vi "initialize.vi"(7 "parameters":string[][](array[string]), 8 "error in":errorcluster, 10 "server id":i32, 11 "message json":string) -> (0 "error out":errorcluster, 3 "response":string)   [LabVIEW 2025, in "MCP Server.lvlib"]
uses:
  MCP Server.lvlib
  098ae85c-509d-4dd3-b755-49cb06aac0fc.vi
  <vilib>/JDP Science/JSONtext/Variant to JSON Text.vi
  <vilib>/JDP Science/JSONtext/LVClass Serializer/JSONtext LVClass Serializer.lvclass
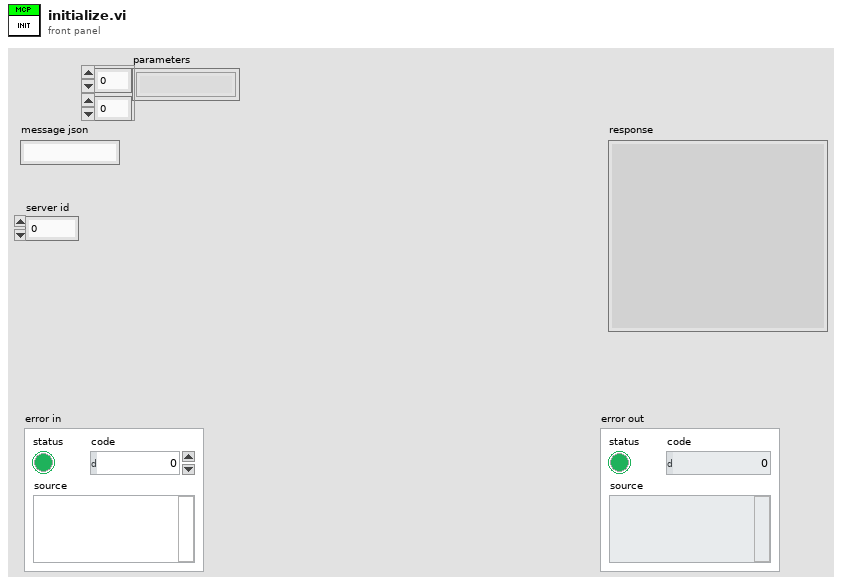
[diagram p1: front panel]
types:
  T1 = cluster{"protocolVersion":string, "capabilities":cluster{"tools":cluster{"listChanged":bool}, "prompts":cluster{"listChanged":bool}, "resources":cluster{"subscribe":bool, "listChanged":bool}}, "serverInfo":cluster{"name":string, "version":string, "additionalDetails":cluster{"labviewVersion":string, "platform":string}}}
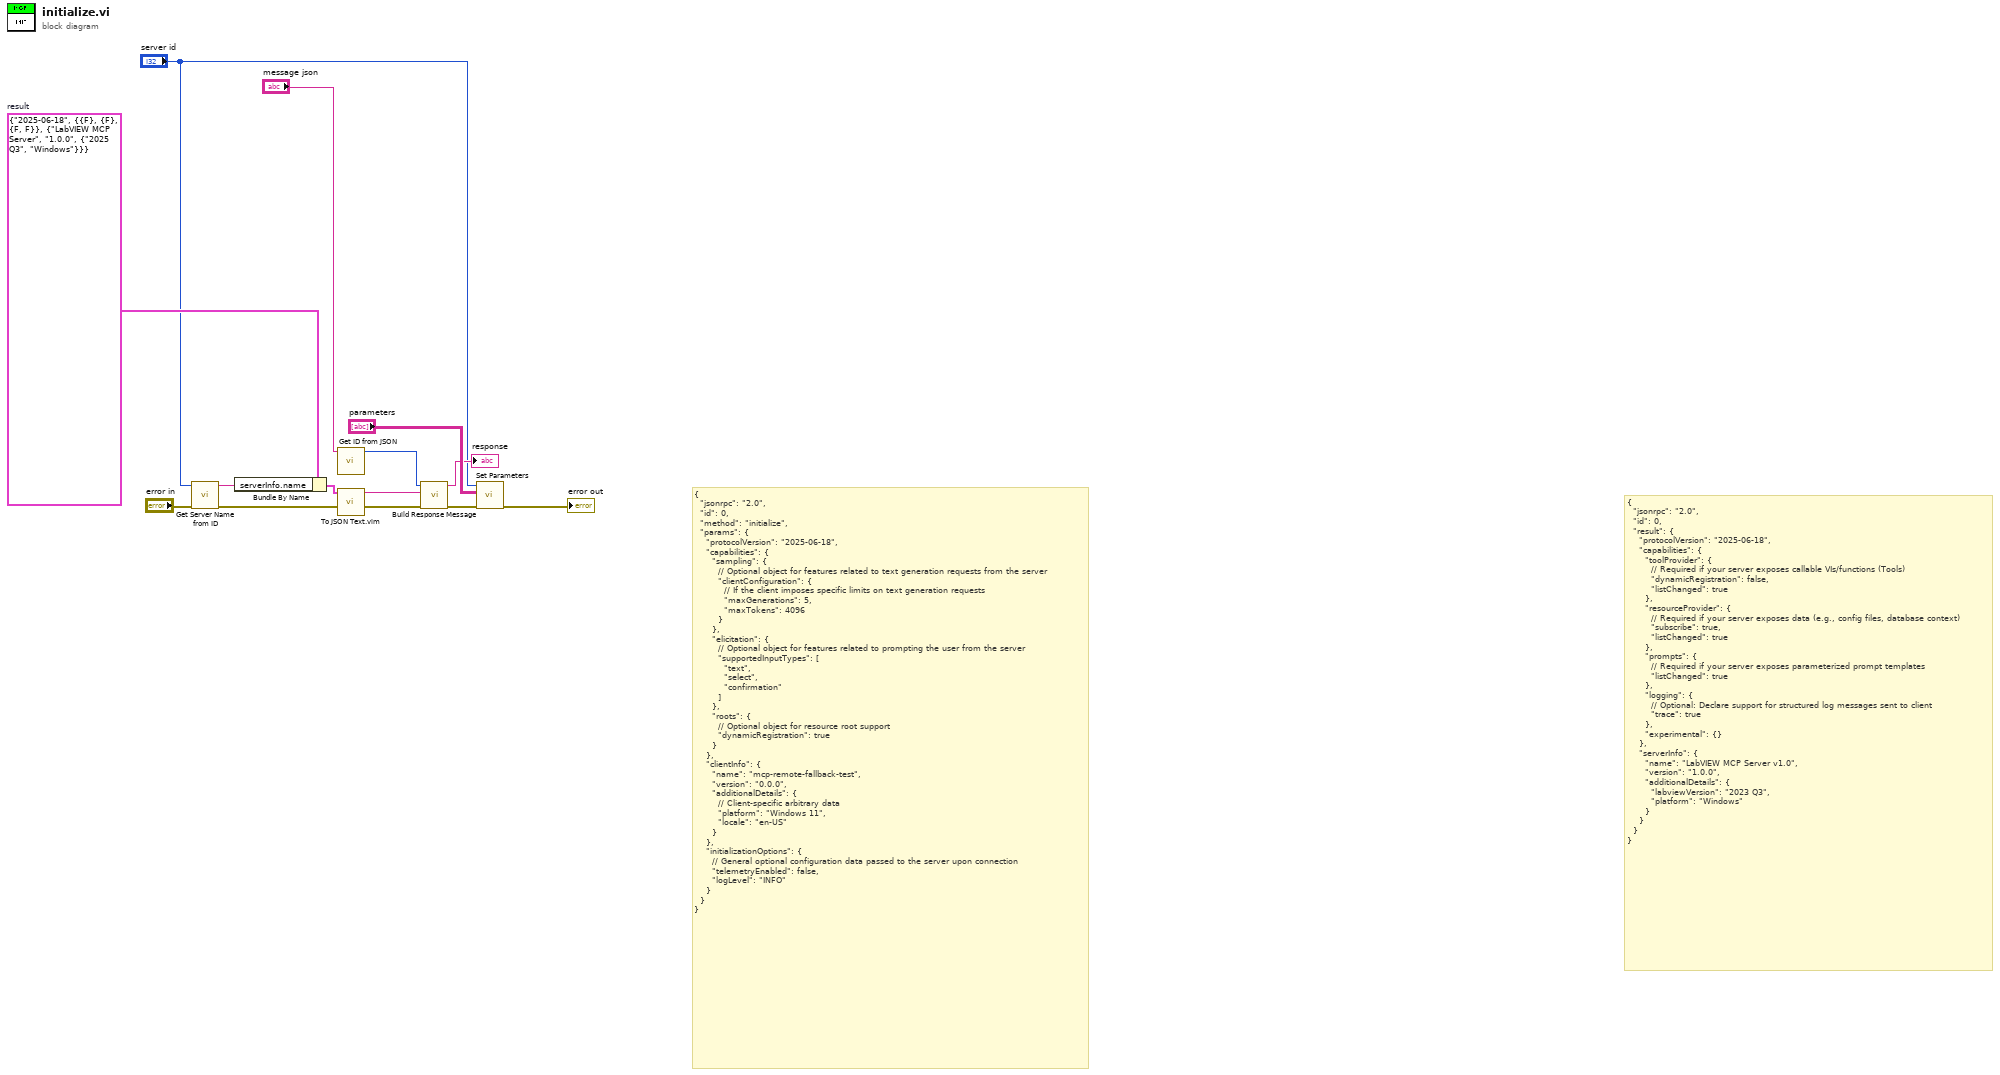
[diagram p0: block diagram]
diagram:
  w9 = T1 {"protocolVersion"="2025-06-18", "capabilities"={"tools"={"listChanged"=FALSE}, "prompts"={"listChanged"=FALSE}, "resources"={"subscribe"=FALSE, "listChanged"=FALSE}}, "serverInfo"={"name"="LabVIEW MCP Server", "version"="1.0.0", "additionalDetails"={"labviewVersion"="2025 Q3", "platform"="Windows"}}}  # result
  # "{\n  \"jsonrpc\": \"2.0\",\n  \"id\": 0,\n  \"method\": \"initialize\",\n  \"params\": {\n    \"protocolVersion\": \"2025-06-18\",\n    \"capabilities\": {\n      \"sampling\": {\n        // Optional object for features related to text generation requests from the server\n        \"clientConfiguration\": {\n          // If the client imposes specific limits on text generation requests\n          \"maxGenerations\": 5,\n          \"maxTokens\": 4096\n        }\n      },\n      \"elicitation\": {\n        // Optional object for features related to prompting the user from the server\n        \"supportedInputTypes\": [\n          \"text\",\n          \"select\",\n          \"confirmation\"\n        ]\n      },\n      \"roots\": {\n        // Optional object for resource root support\n        \"dynamicRegistration\": true\n      }\n    },\n    \"clientInfo\": {\n      \"name\": \"mcp-remote-fallback-test\",\n      \"version\": \"0.0.0\",\n      \"additionalDetails\": {\n        // Client-specific arbitrary data\n        \"platform\": \"Windows 11\",\n        \"locale\": \"en-US\"\n      }\n    },\n    \"initializationOptions\": {\n      // General optional configuration data passed to the server upon connection\n      \"telemetryEnabled\": false,\n      \"logLevel\": \"INFO\"\n    }\n  }\n}"
  # "{\n  \"jsonrpc\": \"2.0\",\n  \"id\": 0,\n  \"result\": {\n    \"protocolVersion\": \"2025-06-18\",\n    \"capabilities\": {\n      \"toolProvider\": {\n        // Required if your server exposes callable VIs/functions (Tools)\n        \"dynamicRegistration\": false,\n        \"listChanged\": true \n      },\n      \"resourceProvider\": {\n        // Required if your server exposes data (e.g., config files, database context)\n        \"subscribe\": true,\n        \"listChanged\": true\n      },\n      \"prompts\": {\n        // Required if your server exposes parameterized prompt templates\n        \"listChanged\": true\n      },\n      \"logging\": {\n        // Optional: Declare support for structured log messages sent to client\n        \"trace\": true\n      },\n      \"experimental\": {}\n    },\n    \"serverInfo\": {\n      \"name\": \"LabVIEW MCP Server v1.0\",\n      \"version\": \"1.0.0\",\n      \"additionalDetails\": {\n        \"labviewVersion\": \"2023 Q3\",\n        \"platform\": \"Windows\"\n      }\n    }\n  }\n}"
  n1 = call "Get Server Name from ID.vi"("error in (no error)"="error in", "id"="server id") -> ("error out"=w1:errorcluster, "name"=w2:string)  [unwired: 8 in]
  n2 = Bundle By Name(cluster=w9, "serverInfo.name"=w2) -> (w4:T1)
  n3 = call "Get ID from JSON.vi"("message json"="message json") -> ("Data out"=w11:i32)  [unwired: 10 in]
  n4 = call "To JSON Text.vim"("error in (no error)"=w1, "Anything"=w4) -> ("error out"=w10:errorcluster, "<JSON>"=w8:string)  [unwired: 8 in]
  n5 = call "Build Response Message.vi"("error in (no error)"=w10, "Result content"=w8, "message id in"=w11) -> ("error out"=w12:errorcluster, "MCP message out"=→"response":string)  [unwired: 7 in]
  n6 = call "Set Parameters.vi"("error in"=w12, "Parameters"="parameters", "id"="server id") -> ("error in 2"=→"error out":errorcluster)  [unwired: 8 in]
